vi "4461 - Create AO waveforms.vi"(9 "sampling info":cluster{"Fs":dbl, "#s":dbl}={"Fs"=1000.0, "#s"=1000.0} {"Fs" format="%.2p"}, 10 "reset signal":bool, 11 "AO":T1={"AO amp (V)"=[0.1, 0.09, 0.08, 0.07, 0.06, 0.05, 0.04, 0.03], "AO DC (V)"=[0.0, 0.0, 0.0, 0.0, 0.0, 0.0, 0.0, 0.0], "AO f (Hz)"=[13.0, 13.0, 13.0, 13.0, 13.0, 13.0, 13.0, 13.0], "AO phi (deg)"=[0.0, 0.0, 0.0, 0.0, 0.0, 0.0, 0.0, 0.0], "function"=[enum."Sine Wave", enum."Sine Wave", enum."Sine Wave", enum."Sine Wave", enum."Sine Wave", enum."Sine Wave", enum."Sine Wave", enum."Sine Wave"]} {"AO DC (V)" format="%#_6p"; "AO amp (V)" format="%#_6p"}) -> (0 "phase out":dbl[](array[numeric]), 1 "AO Array":waveform(dbl)[](array[waveform]), 3 "AO 2":T1={"AO amp (V)"=[0.1, 0.09, 0.08, 0.07, 0.06, 0.05, 0.04, 0.03], "AO DC (V)"=[0.0, 0.0, 0.0, 0.0, 0.0, 0.0, 0.0, 0.0], "AO f (Hz)"=[13.0, 13.0, 13.0, 13.0, 13.0, 13.0, 13.0, 13.0], "AO phi (deg)"=[0.0, 0.0, 0.0, 0.0, 0.0, 0.0, 0.0, 0.0], "function"=[enum."Sine Wave", enum."Sine Wave", enum."Sine Wave", enum."Sine Wave", enum."Sine Wave", enum."Sine Wave", enum."Sine Wave", enum."Sine Wave"]} {"AO DC (V)" format="%#_6p"; "AO amp (V)" format="%#_6p"})   [LabVIEW 2013]
uses:
  <vilib>/Analysis/2dsp.llb/Decimate (single shot).vi
  <vilib>/Analysis/2dsp.llb/Decimate (single shot, DBL).vi
  <vilib>/Utility/error.llb/Error Cluster From Error Code.vi
  <vilib>/measure/NI_MABase.lvlib
panel:
  out "Waveform Graph 2":waveform(dbl)[](graph)=[{"t0"=timestamp(0 s since 1904-01-01), "dt"=4.8828125e-06, "Y"=array[20480 elements]}, {"t0"=timestamp(0 s since 1904-01-01), "dt"=4.8828125e-06, "Y"=array[20480 elements]}, {"t0"=timestamp(0 s since 1904-01-01), "dt"=4.8828125e-06, "Y"=array[20480 elements]}, {"t0"=timestamp(0 s since 1904-01-01), "dt"=4.8828125e-06, "Y"=array[20480 elements]}, {"t0"=timestamp(0 s since 1904-01-01), "dt"=4.8828125e-06, "Y"=array[20480 elements]}, {"t0"=timestamp(0 s since 1904-01-01), "dt"=4.8828125e-06, "Y"=array[20480 elements]}, {"t0"=timestamp(0 s since 1904-01-01), "dt"=4.8828125e-06, "Y"=array[20480 elements]}, {"t0"=timestamp(0 s since 1904-01-01), "dt"=4.8828125e-06, "Y"=array[20480 elements]}]
  out "Numeric":i32
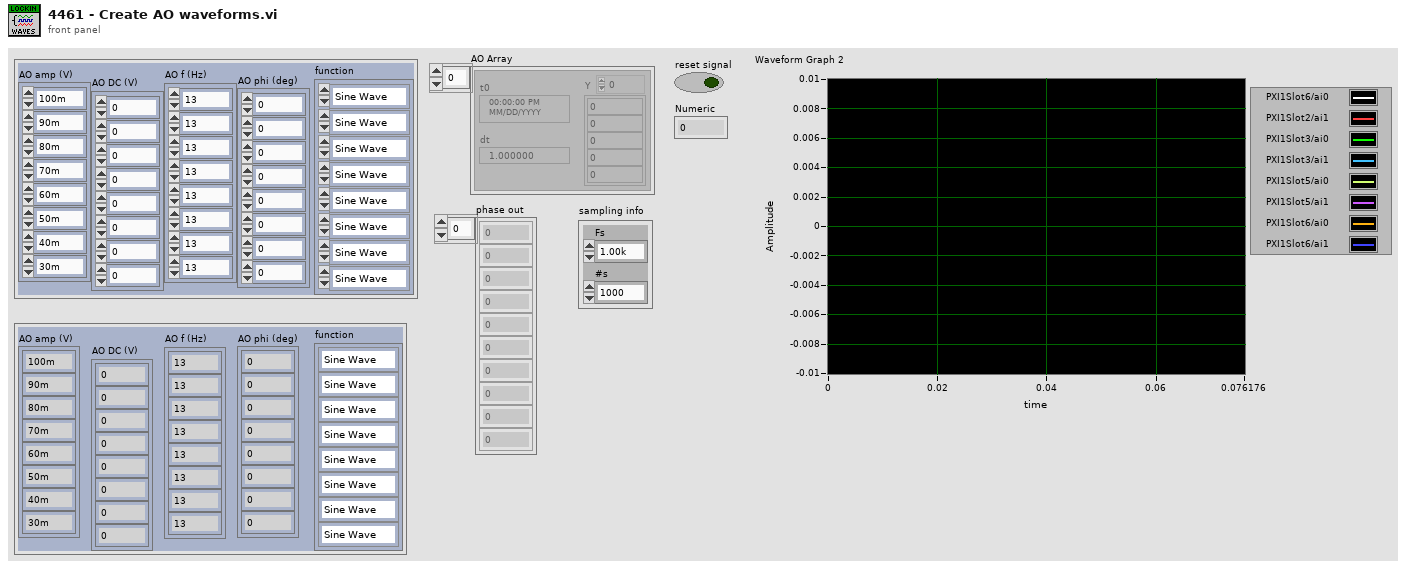
[diagram p1: front panel]
types:
  T1 = cluster{"AO amp (V)":dbl[], "AO DC (V)":dbl[], "AO f (Hz)":dbl[], "AO phi (deg)":dbl[], "function":enum16{"Sine Wave", "Triangle Wave", "Square Wave", "Sawtooth Wave"}[]}
  T2 = enum16{"Sine Wave", "Triangle Wave", "Square Wave", "Sawtooth Wave"}[]
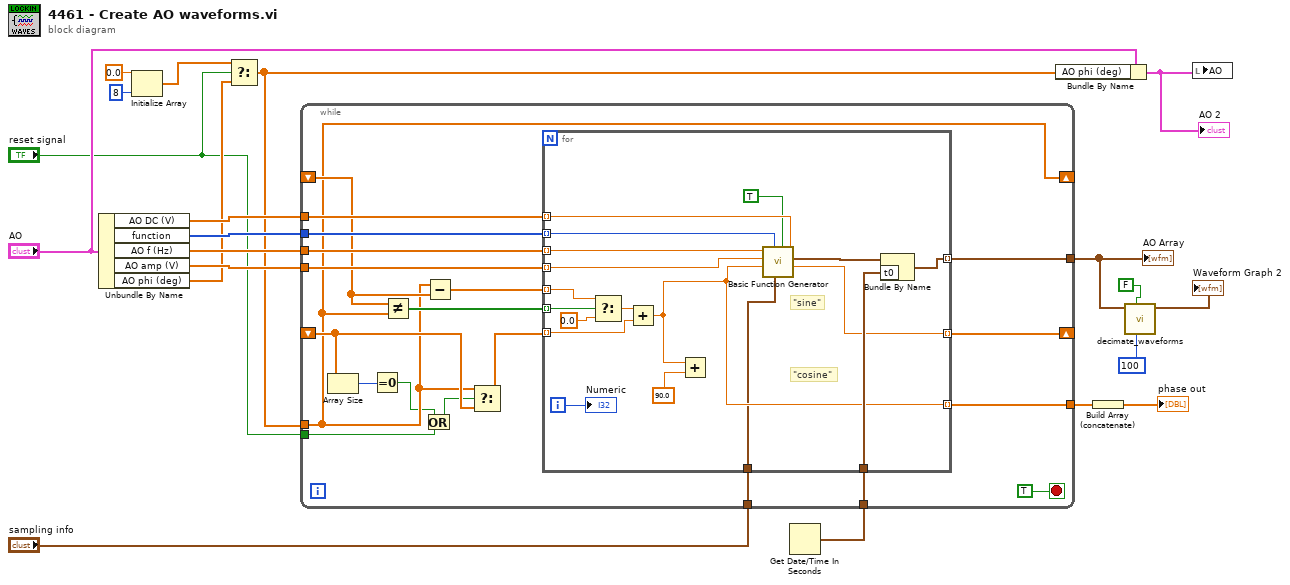
[diagram p0: block diagram]
diagram:
  n1 = Unbundle By Name("AO") -> ("AO DC (V)"=w19:dbl[], "function"=w20:T2, "AO f (Hz)"=w16:dbl[], "AO amp (V)"=w17:dbl[], "AO phi (deg)"=w9:dbl[])
  n2 = Initialize Array(0.0 ("element"), 8 ("dimension size")) -> (w10:dbl[])
  n3 = Select(t=w10, s="reset signal", f=w9) -> (s? t:f=w8:dbl[])
  n4 = Get Date/Time In Seconds() -> (seconds since 1Jan1904=w13:timestamp)
  n5 = while {
    tunnel: w20 -> [w40]
    tunnel: w19 -> [w39]
    tunnel: "sampling info" -> [w38]
    tunnel: [w37] -> w2
    tunnel: w17 -> [w36]
    tunnel: w8 -> [w26]
    tunnel: w16 -> [w35]
    shift-right: [w26] -> _
    shift-left: _ -> [w32]
    shift-right: [w30] -> _
    shift-left: _ -> [w28]
    tunnel: w13 -> [w29]
    tunnel: "reset signal" -> [w23]
    tunnel: [w22] -> w6
    stop <- TRUE stop-if-true
    n6 = Array Size(array=w28) -> (size(s)=w27:i32)
    n7 = Equal To 0?(x=w27) -> (x = 0?=w24:bool)
    n8 = Not Equal?(x=w32, y=w26) -> (x != y?=w33:bool[])
    n9 = Or(x=w24, y=w23) -> (x .or. y?=w25:bool)
    n10 = Subtract(x=w26, y=w32) -> (x-y=w31:dbl[])
    n11 = Select(t=w26, s=w25, f=w28) -> (s? t:f=w21:dbl[])
    n12 = for {
      tunnel: w40 -> [w58] mode=indexing
      tunnel: w35 -> [w57] mode=indexing
      tunnel: w36 -> [w56] mode=indexing
      tunnel: w39 -> [w55] mode=indexing
      tunnel: [w41] -> w37 mode=indexing
      tunnel: w38 -> [w43]
      tunnel: w33 -> [w48] mode=indexing
      tunnel: w31 -> [w50] mode=indexing
      tunnel: [w42] -> w30 mode=indexing
      tunnel: w21 -> [w51] mode=indexing
      tunnel: w29 -> [w47]
      tunnel: [w44] -> w22 mode=indexing
      i -> [w46]
      # "\"cosine\""
      # "\"sine\""
      n13 = Select(t=w50, s=w48, f=0.0) -> (s? t:f=w52:dbl)
      n14 = Add(x=w52, y=w51) -> (x+y=w44:dbl)
      n15 = Add(x=w44, y=90.0) -> ()  [unwired: 1 out]
      n16 = call <vilib>:"Basic Function Generator.vi"("offset"=w55, "reset signal"=TRUE, "sampling info"=w43, "signal type"=w58, "phase"=w44, "amplitude"=w56, "frequency"=w57) -> ("phase out"=w42:dbl, "signal out"=w54:waveform(dbl))  [unwired: 2 in, 1 out]
      n17 = Bundle By Name(cluster=w54, "t0"=w47) -> (w41:waveform(dbl))
      "Numeric" <- w46
    }
  }
  "AO Array" <- w2
  n18 = Bundle By Name(cluster="AO", "AO phi (deg)"=w8) -> (w11:T1)
  "AO 2" <- w11
  n19 = Build Array (concatenate)(w6) -> (→"phase out":dbl[])
  n20 = call "decimate_waveforms.vi"("decimating factor"=100, "averaging"=FALSE, "Input Signal"=w2) -> ("Decimated Waveforms"=→"Waveform Graph 2":waveform(dbl)[])  [unwired: 7 in, 1 out]
  n21 = local write "AO"(w11) -> ()
